vi "MSScript_Act_ExportResults.vi"(7 "user param refnum":refnum<vi>, 8 "error in (no error)":errorcluster, 11 "MSScript in":refnum<class "MSScript.lvclass">) -> (0 "error out":errorcluster, 1 "Ion trap":cluster{"R0":ext, "Z0":ext}, 2 "PriRF":T2, 3 "MS Process fmts":cluster{"Name":string, "Data":variant}[](array[cluster]), 5 "Script out":T1)   [LabVIEW 2018, in "MSScript.lvclass"]
uses:
  MSScript.lvclass
  MSScript.lvclass/MSScript.ctl
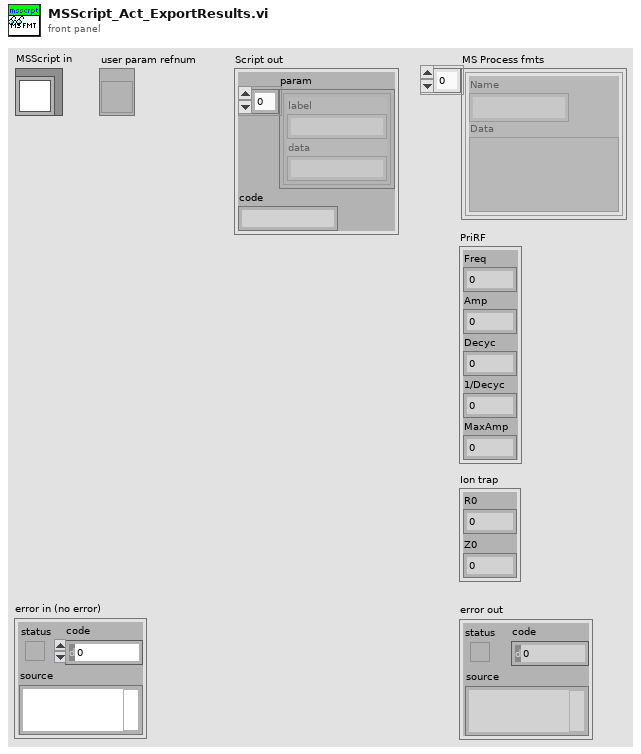
[diagram p1: front panel]
types:
  T1 = cluster{"param":cluster{"label":string, "data":string}[], "code":string}
  T2 = cluster{"Freq":ext, "Amp":ext, "Decyc":u32, "1/Decyc":u32, "MaxAmp":ext}
  T3 = enum8{"Enabled", "Disabled", "Disabled and Grayed Out"}
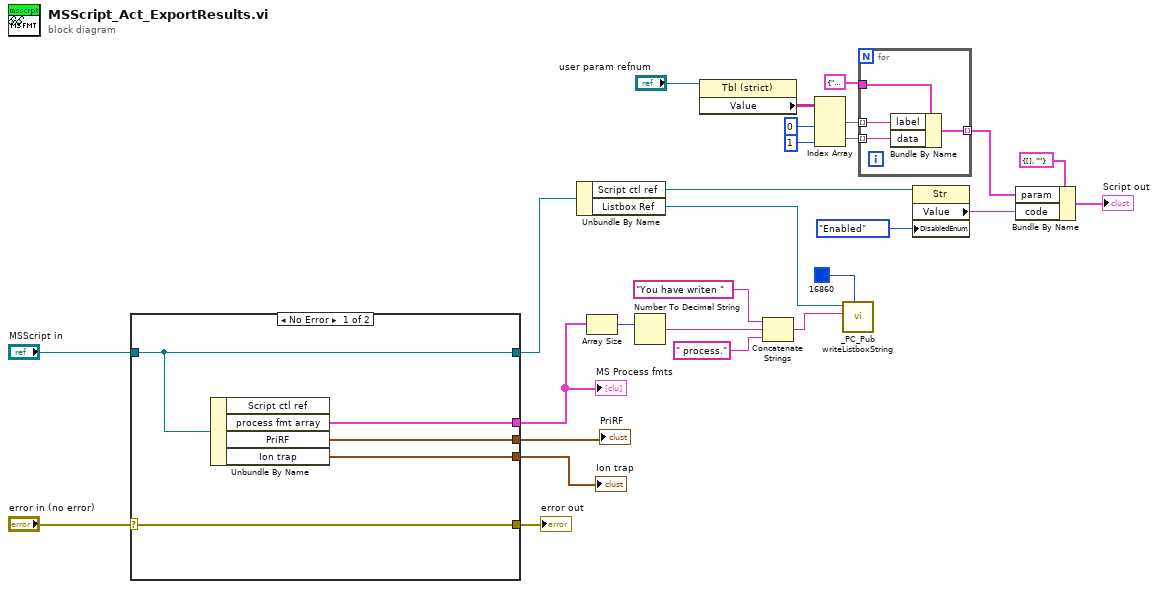
[diagram p0: block diagram]
diagram:
  n1 = case shown="No Error" "error in (no error)" {
    selector: "error in (no error)" -> [w32 w33]
    tunnel: [w32 w33] -> w26
    tunnel: [w31 w34] -> w21
    tunnel: "MSScript in" -> [w31 w34]
    tunnel: [w30 _] -> w19
    tunnel: [w29 _] -> w24
    tunnel: [w28 _] -> w23
    frame No Error {
      n2 = Unbundle By Name(w31) -> ("process fmt array"=w30:cluster{"Name":string, "Data":variant}[], "PriRF"=w29:T2, "Ion trap"=w28:cluster{"R0":ext, "Z0":ext})  [unwired: 1 out]
    }
    frame Error {
    }
  }
  "error out" <- w26
  "MS Process fmts" <- w19
  "Ion trap" <- w23
  "PriRF" <- w24
  n3 = Unbundle By Name(w21) -> ("Script ctl ref"=w20:refnum<vi>, "Listbox Ref"=w17:refnum<vi>)
  n4 = Array Size(array=w19) -> (size(s)=w18:i32)
  n5 = Number To Decimal String(number=w18) -> (decimal integer string=w16:string)  [unwired: 1 in]
  n6 = property class="Tbl (strict)"(reference="user param refnum") -> ("Value"=w2:string[][])  [unwired: 1 in, 2 out]
  n7 = Concatenate Strings("You have writen " ("string"), w16, " process." ("string")) -> (w13:string)
  n8 = Index Array(array=w2, index (col) #1=0 ("disabled index (col)"), index (col) #2=1 ("index (col)")) -> (element #1=w6:string[], element #2=w7:string[])  [unwired: 2 in]
  n9 = call "_PC_Pub writeListboxString.vi"("String Color"=u32 16860, "update_Str"=w13, "Listbox Ref Input"=w17) -> ()  [unwired: 7 in, 2 out]
  n10 = for {
    tunnel: w6 -> [w37] mode=indexing
    tunnel: w7 -> [w36] mode=indexing
    tunnel: cluster{"label":string, "data":string} {"label"="", "data"=""} -> [w38]
    tunnel: [w35] -> w1 mode=indexing
    n11 = Bundle By Name(cluster=w38, "label"=w37, "data"=w36) -> (w35:cluster{"label":string, "data":string})
  }
  n12 = property class="Str"(reference=w20, "DisabledEnum"=T3."Enabled" ("Disabled")) -> ("Value"=w10:string)  [unwired: 1 in, 2 out]
  n13 = Bundle By Name(cluster=T1 {"param"=[], "code"=""} ("Script out"), "param"=w1, "code"=w10) -> (→"Script out":T1)
